vi "sub1.vi"(10 "클러스터":cluster{"오백원 갯수":i32, " 백원 갯수":i32}, 11 "클러스터 2":cluster{"잔여금액":i32, "카드결제\n금액":i32, "음료가격":i32}) -> (1 "숫자형":i32, 2 "숫자형 2":i32, 3 "불리언 2":bool, 4 "오백원 갯수":i32, 5 "불리언":bool, 6 "불리언 3":bool)   [LabVIEW 2016]
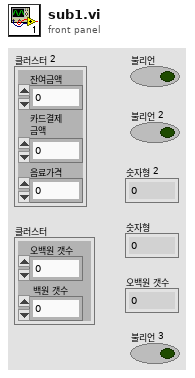
[diagram p1: front panel]
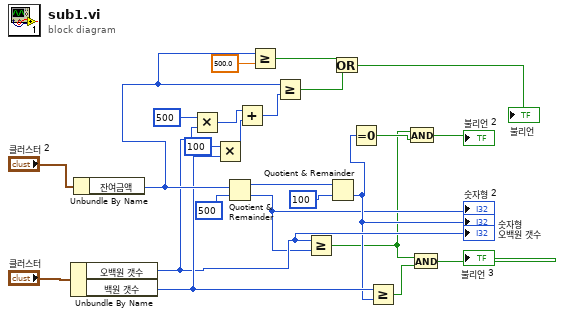
[diagram p0: block diagram]
diagram:
  n1 = Unbundle By Name("클러스터") -> ("오백원 갯수"=w11:i32, "백원 갯수"=w14:i32)
  "오백원 갯수" <- w11
  n2 = Unbundle By Name("클러스터 2") -> ("잔여금액"=w21:i32)
  n3 = Multiply(x=500, y=w11) -> (x*y=w16:i32)
  n4 = Multiply(x=100, y=w14) -> (x*y=w15:i32)
  n5 = Quotient & Remainder(x=w21, y=500) -> (x-y*floor(x/y)=w5:i32, floor(x/y)=w9:i32)
  "숫자형 2" <- w9
  n6 = Add(x=w16, y=w15) -> (x+y=w17:i32)
  n7 = Greater Or Equal?(x=w21, y=500.0) -> (x >= y?=w22:bool)
  n8 = Greater Or Equal?(x=w21, y=w17) -> (x >= y?=w23:bool)
  n9 = Greater Or Equal?(x=w11, y=w9) -> (x >= y?=w7:bool)
  n10 = Quotient & Remainder(x=w5, y=100) -> (floor(x/y)=w10:i32)  [unwired: 1 out]
  "숫자형" <- w10
  n11 = Or(x=w22, y=w23) -> (x .or. y?=→"불리언":bool)
  n12 = Equal To 0?(x=w10) -> (x = 0?=w18:bool)
  n13 = Greater Or Equal?(x=w14, y=w10) -> (x >= y?=w8:bool)
  n14 = And(x=w7, y=w18) -> (x .and. y?=→"불리언 2":bool)
  n15 = And(x=w7, y=w8) -> (x .and. y?=→"불리언 3":bool)
